vi "read_raw_dataV3.0_timestamp.vi"() -> ()   [LabVIEW 2017]
uses:
  <vilib>/Utility/file.llb/Read Delimited Spreadsheet (I64).vi
  <vilib>/Utility/file.llb/Write Delimited Spreadsheet (DBL).vi
  <vilib>/Utility/file.llb/Write Delimited Spreadsheet (I64).vi
  <vilib>/Utility/file.llb/Write Delimited Spreadsheet (string).vi
panel:
  out "offset past number 3":i32=1
  out "offset past number 2":i32=46
  out "offset past number":i32=15
  out "hex integer string 2":string="15"
  out "hex integer string":string="1"
  out "substring 5":string
  out "substring 4":string
  out "substring 3":string="."
  out "substring 2":string="46"
  out "output 1":timestamp=timestamp(3800538946 s since 1904-01-01)
  in  "output 4":timestamp=timestamp(3800536645.628 s since 1904-01-01)
  out "Numeric":dbl=-33699.628
  in  "date/time string 4":string="  6/7/2024"
  out "date/time string 3":string="1:15:46  6/7/2024"
  in  "col":i32
  in  "file path (dialog if empty)":path=path "G:/tdc/2017/code_density_rom.mem"
  out "size(s)":i32[](array[numeric])=[2048, 128]
  out "Array":u32[][](array[numeric]) format="%x"
  out "cal":u32[][](graph)
  out "x/y":dbl=0.0025
  out "index":i32=1018
  out "time":dbl=636682692500.0 format="%.000f"
  in  "通道数量":i32=128
  out "fine":u64=356 format="%x"
  out "data 5":string
  in  "ch list":u16[](array[numeric])=[0, 1, 2, 3, 4, 5, 6, 7]
  in  "codeDensity":path=path "G:/tdc/2017/test_20240607_060014_codeDensity.csv"
  out "file path (dialog if empty) 2":path=path "G:/tdc/2017/test_20240607_060014.txt"
  out "ip":u64=35 format="%x"
  out "data 9":string="#"
  out "result string":string="test_20240607_060014"
  out "sent number":u64=1000 format="%x"
  out "trigger number":u64=257 format="%x"
  out "data 8":string
  out "data 7":string
  out "data":u64[](array[numeric])=[35, 1, 1000, 257, 41715683595775000] format="%x"
  out "data 2":string
  out "data 4":string
  out "coarse time":u64=254673077 format="%x"
  out "error out":errorcluster
  out "substring":string=""
  out "number 3":u32
  out "channel number":u64=1 format="%x"
  in  "channel":u64
  out "data 6":string
  out "data 3":string="Z"
  in  "dat file (use dialog)":path=path "G:/tdc/2017/test_20240607_060014.dat"
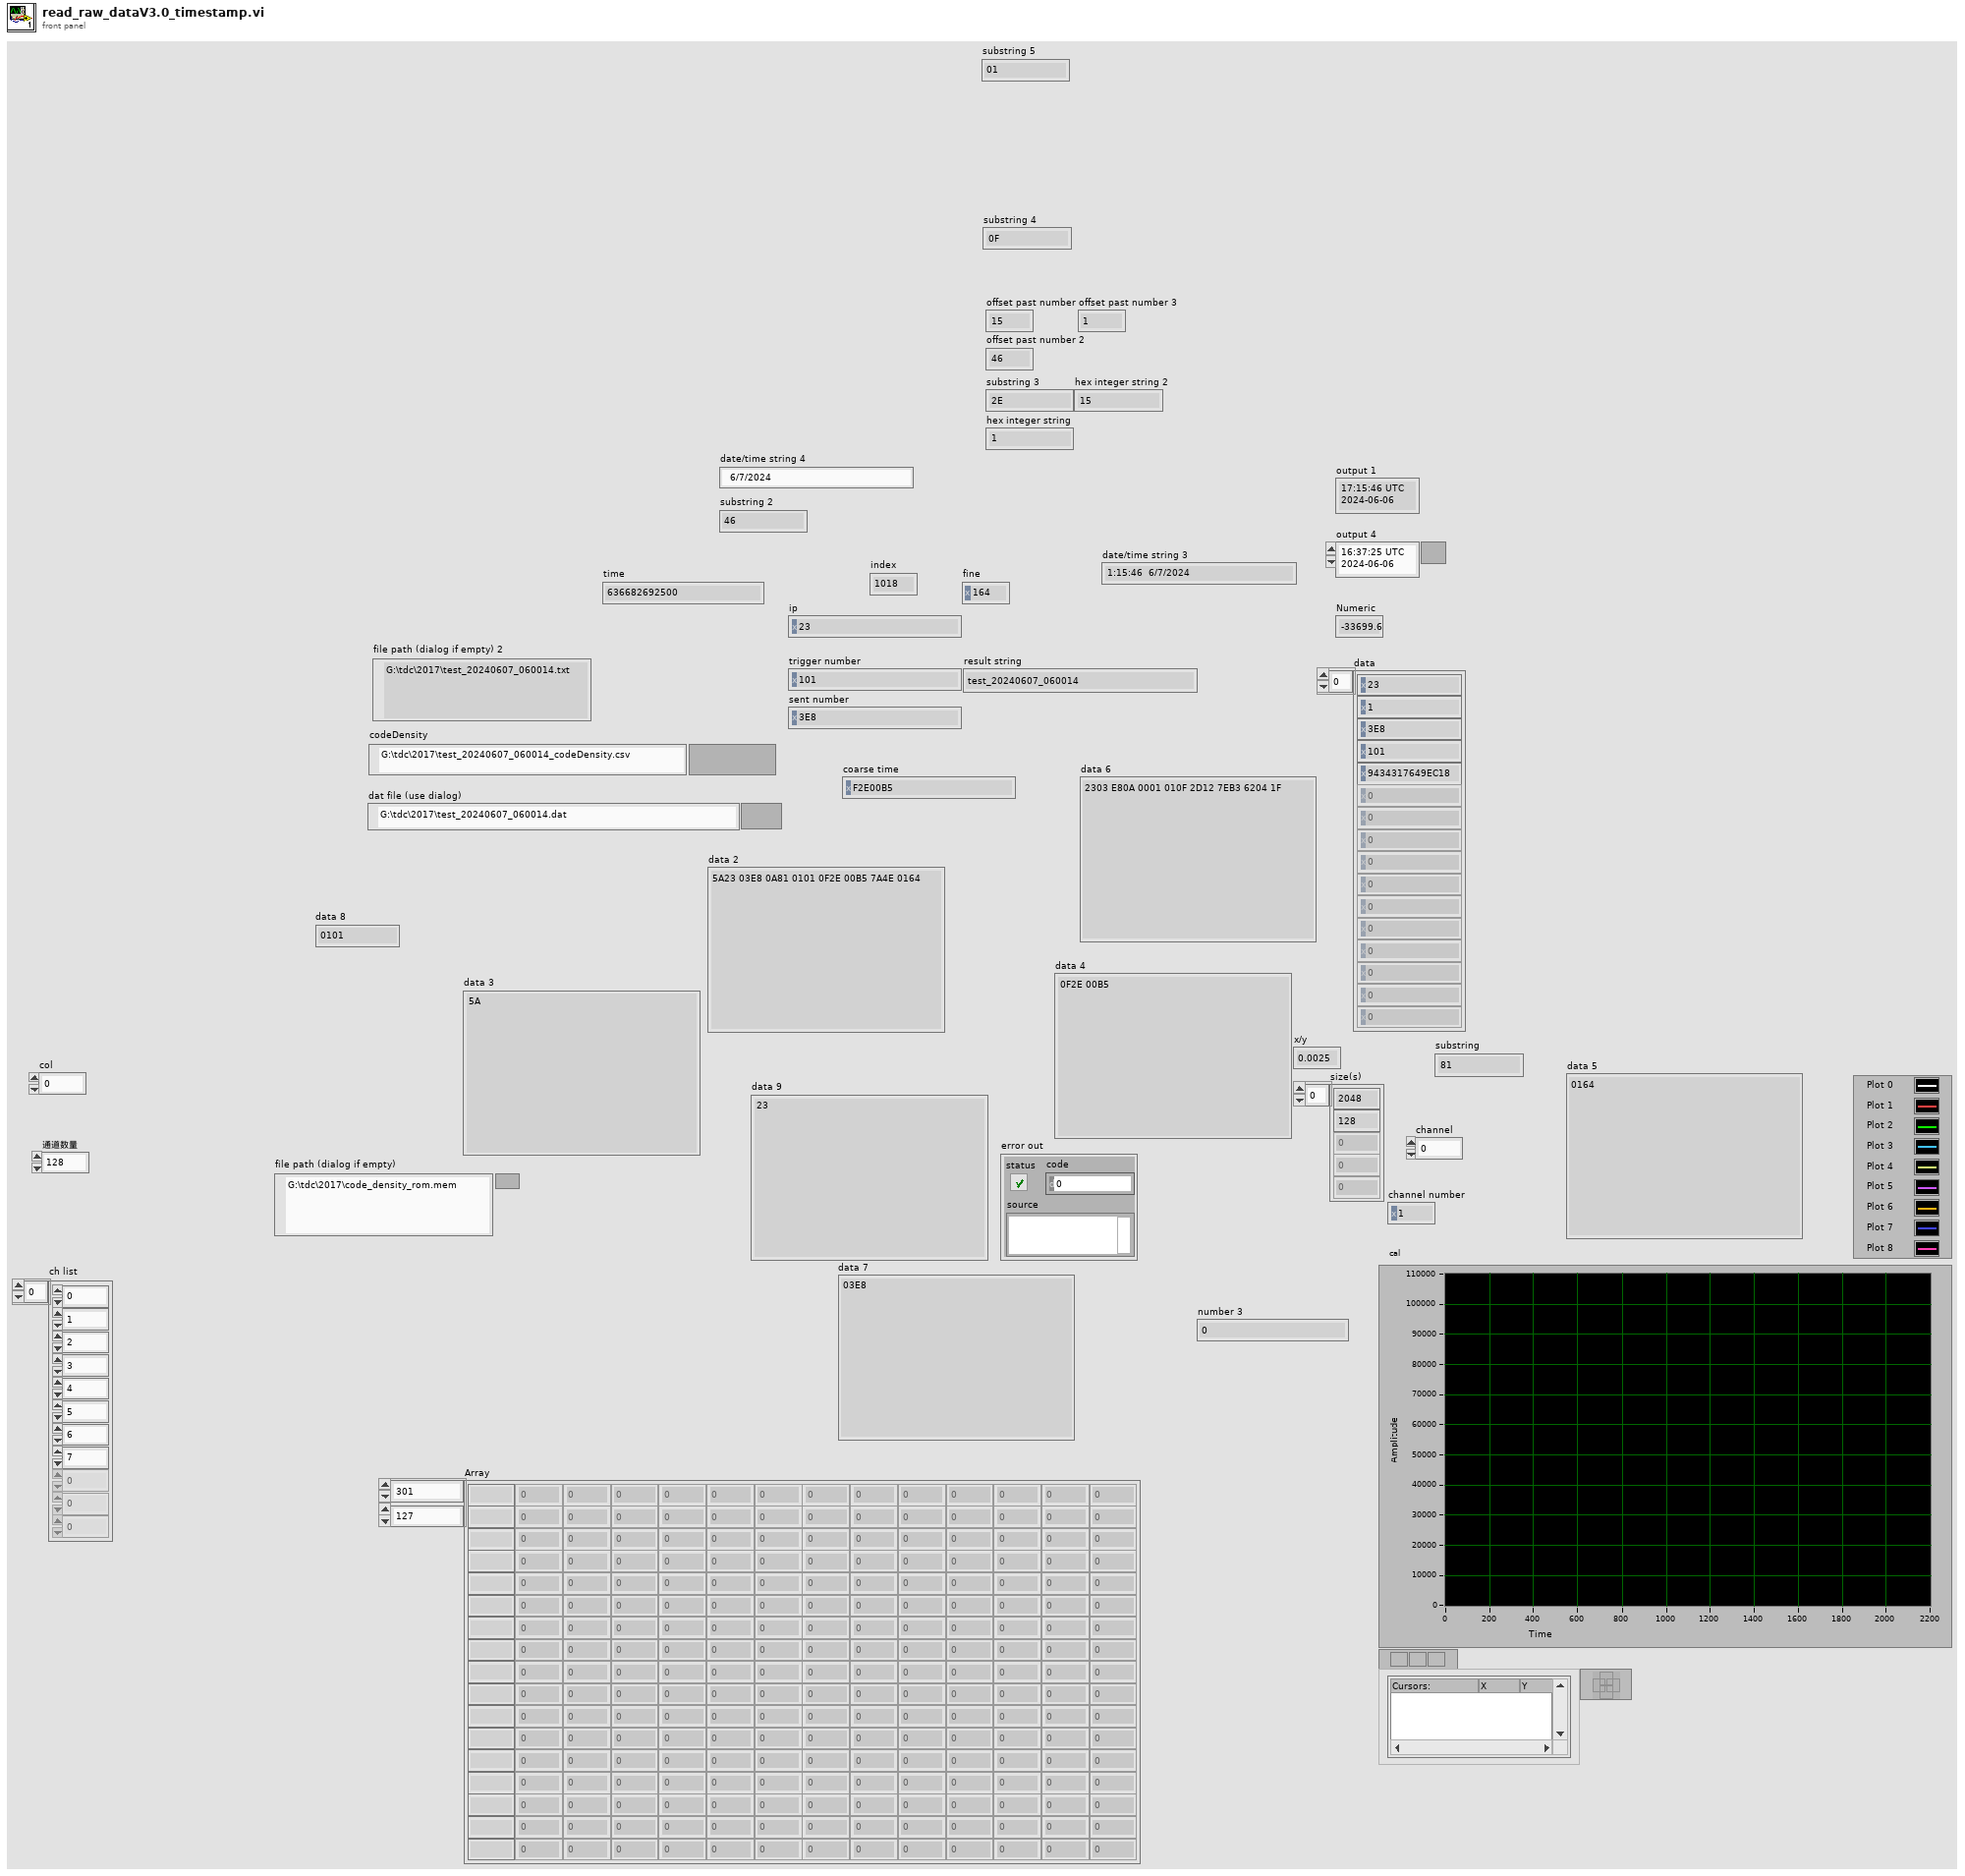
[diagram p1: front panel]
types:
  T1 = enum16{"open", "replace", "create", "open or create", "replace or create", "replace or create with confirmation"}
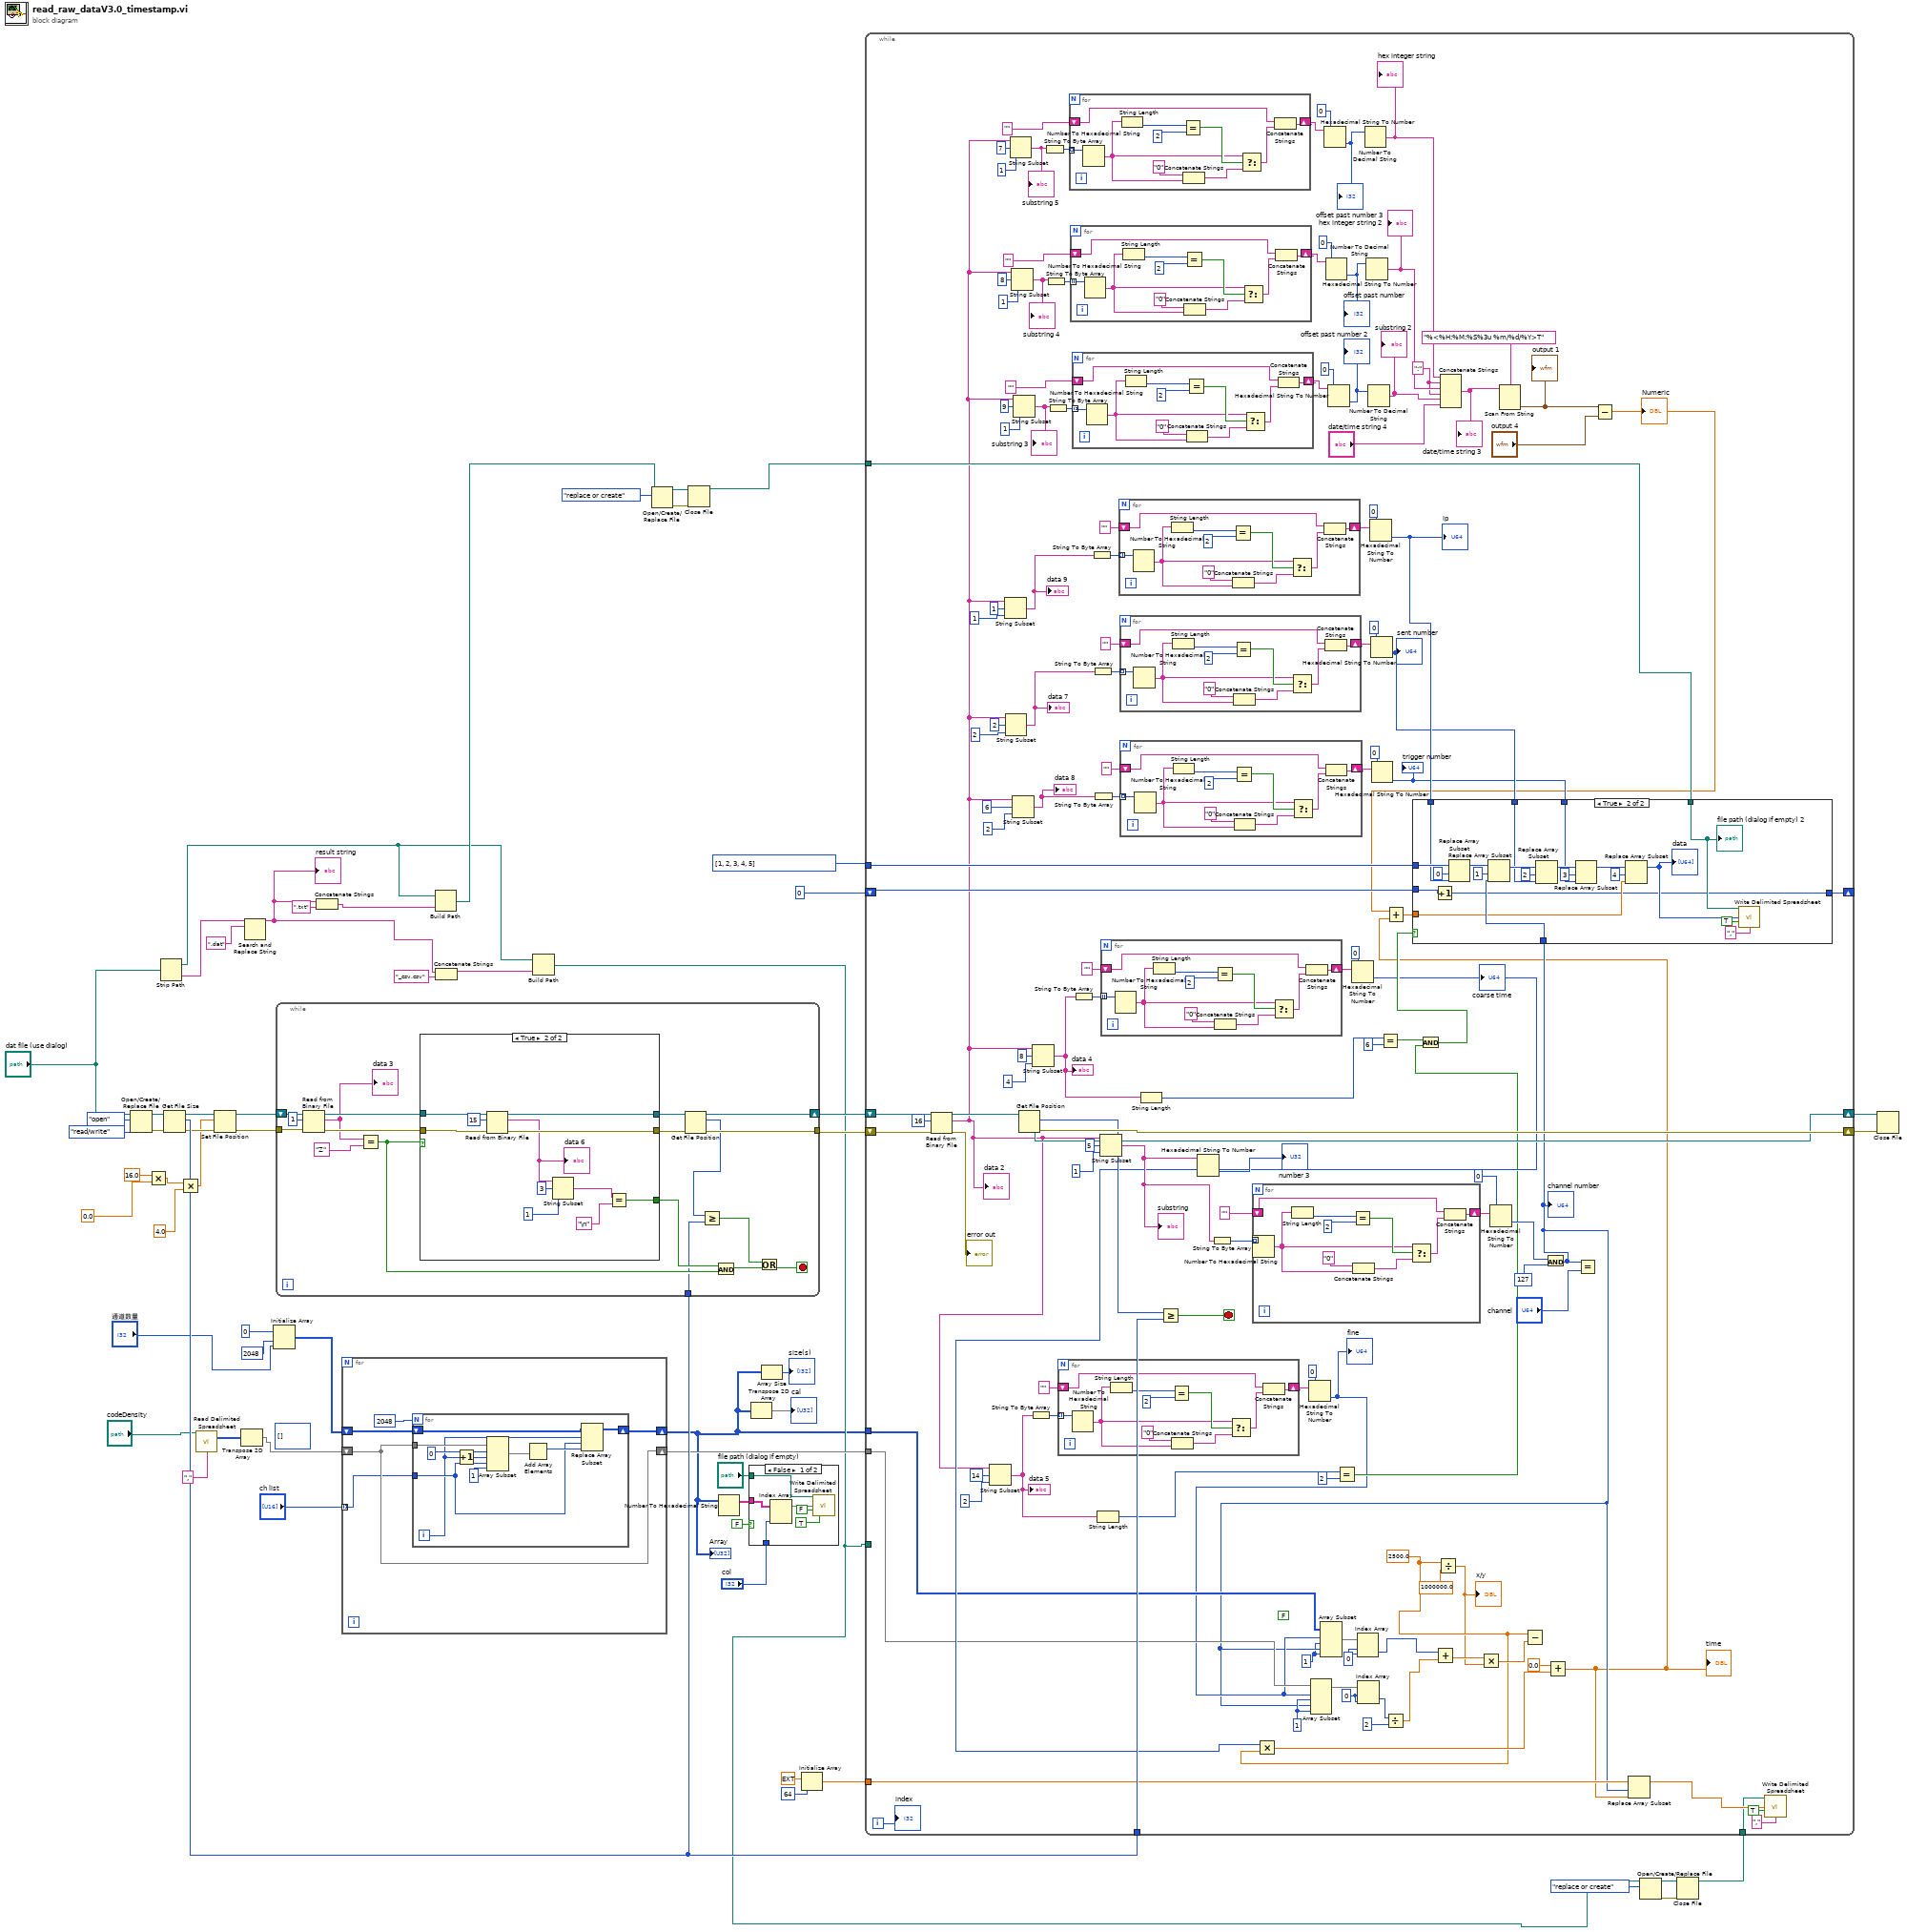
[diagram p0: block diagram]
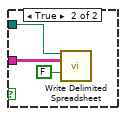
[diagram p2: hidden frame]
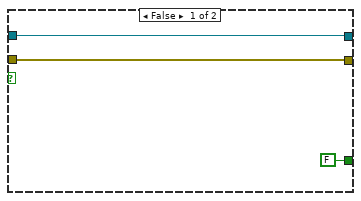
[diagram p4: hidden frame]
diagram:
  (unwired) i64[][] []
  n1 = Open/Create/Replace File(file path (use dialog)="dat file (use dialog)", operation (0:open)=T1."open", access (0:read/write)=enum16{"read/write", "read-only", "write-only"}."read/write") -> (refnum out=w59:refnum<file>, error out=w54:errorcluster)  [unwired: 3 in, 1 out]
  n2 = Multiply(x=16.0, y=0.0) -> (x*y=w20:dbl)
  n3 = Strip Path(path="dat file (use dialog)") -> (stripped path=w9:path, name=w47:string)
  n4 = Get File Size(file=w59, error in=w54) -> (refnum out=w26:refnum<file>, size (in bytes)=w49:i64, 0:w24:errorcluster)
  n5 = Multiply(x=w20, y=4.0) -> (x*y=w18:dbl)
  n6 = call-poly <vilib>:"Read Delimited Spreadsheet.vi"("file path (dialog if empty)"="codeDensity", "delimiter (\\t)"="," ("delimiter (\\t)")) -> ("all rows"=w43:i64[][])  [unwired: 8 in, 5 out]
  n7 = Set File Position(offset (in bytes) (0)=w18, refnum=w26, error in=w24) -> (refnum out=w25:refnum<file>, error out=w23:errorcluster)  [unwired: 1 in]
  n8 = Transpose 2D Array(2D array=w43) -> (transposed array=w31:i64[][])
  n9 = Search and Replace String(input string=w47, search string=".dat") -> (result string=w11:string)  [unwired: 6 in, 3 out]
  "result string" <- w11
  n10 = Initialize Array(u32 0 ("element"), 2048 ("dimension size"), "通道数量") -> (w32:u32[][])
  n11 = while {
    tunnel: w23 -> [w76]
    shift-right: [w64] -> w55
    shift-left: w25 -> [w77]
    tunnel: [w65] -> w56
    tunnel: w49 -> [w63]
    stop <- w61 stop-if-true
    n12 = Read from Binary File(8:w76, 10:1 ("count (1)"), 11:w77) -> (0:w72:errorcluster, 2:w70:string, 3:w73:refnum<file>)  [unwired: 3 in, 1 out]
    "data 3" <- w70
    n13 = Equal?(x=w70, y="Z") -> (x = y?=w67:bool)
    n14 = case shown="True" w67 {
      tunnel: w73 -> [w80 w91]
      tunnel: w72 -> [w79 w90]
      tunnel: [w80 w88] -> w71
      tunnel: [w79 w87] -> w66
      tunnel: [FALSE w81] -> w68
      frame False {
      }
      frame True {
        n15 = Read from Binary File(8:w90, 10:15 ("count (1)"), 11:w91) -> (0:w87:errorcluster, 2:w84:string, 3:w88:refnum<file>)  [unwired: 3 in, 1 out]
        "data 6" <- w84
        n16 = String Subset(string=w84, offset (0)=3, length (rest)=1 ("length (rest)")) -> (substring=w83:string)
        n17 = Equal?(x=w83, y="\n") -> (x = y?=w81:bool)
      }
    }
    n18 = Get File Position(4:w66, 7:w71) -> (0:w65:errorcluster, 2:w62:i64, 3:w64:refnum<file>)
    n19 = Greater Or Equal?(x=w62, y=w63) -> (x >= y?=w60:bool)
    n20 = Compound Arithmetic op=AND(w68, w67) -> (w69:bool)
    n21 = Or(x=w60, y=w69) -> (x .or. y?=w61:bool)
  }
  n22 = Concatenate Strings(w11, ".txt" ("string")) -> (w44:string)
  n23 = for {
    shift-right: [w94] -> w4
    shift-left: w32 -> [w95]
    shift-right: [w93] -> w39
    shift-left: w31 -> [w93]
    tunnel: "ch list" -> [w92] mode=indexing
    n24 = for {
      N: 2048 -> [_]
      tunnel: w93 -> [w106]
      tunnel: w92 -> [w99]
      shift-right: [w101] -> w94
      shift-left: w95 -> [w102]
      i -> [w98]
      n25 = Increment(x=w98) -> (x+1=w97:i32)
      n26 = Array Subset(array=w106, index (row)=0 ("索引"), length (row)=w97, index (col)=w99, length (col)=1 ("长度")) -> (w103:i64[][])
      n27 = Add Array Elements(numeric array=w103) -> (sum=w100:i64)
      n28 = Replace Array Subset(array=w102, new element=w100, index (row)=w98, index (col)=w99) -> (w101:u32[][])
    }
  }
  "Array" <- w4
  n29 = Build Path(base path=w9, name or relative path=w44) -> (appended path=w14:path)
  n30 = Concatenate Strings(w11, "_csv.csv" ("string")) -> (w10:string)
  n31 = Build Path(base path=w9, name or relative path=w10) -> (appended path=w8:path)
  n32 = Open/Create/Replace File(file path (use dialog)=w14, operation (0:open)=T1."replace or create") -> (refnum out=w15:refnum<file>, error out=w16:errorcluster)  [unwired: 4 in, 1 out]
  n33 = Close File(refnum=w15, error in=w16) -> (path=w13:path)  [unwired: 1 out]
  n34 = Number To Hexadecimal String(2:w4) -> (0:w3:string[][])  [unwired: 1 in]
  n35 = case shown="False" FALSE {
    tunnel: "file path (dialog if empty)" -> [w111 w115]
    tunnel: w3 -> [w110 w113]
    tunnel: "col" -> [w108 _]
    frame False {
      n36 = Index Array(array=w110, index (col)=w108) -> (element=w109:string[])  [unwired: 1 in]
      n37 = call-poly <vilib>:"Write Delimited Spreadsheet.vi"("file path (dialog if empty)"=w111, "1D data"=w109, "append to file? (new file:F)"=FALSE, "transpose? (no:F)"=TRUE) -> ()  [unwired: 10 in, 2 out]
    }
    frame True {
      n38 = call-poly <vilib>:"Write Delimited Spreadsheet.vi"("file path (dialog if empty)"=w115, "2D data"=w113, "append to file? (new file:F)"=FALSE) -> ()  [unwired: 11 in, 2 out]
    }
  }
  n39 = Transpose 2D Array(2D array=w4) -> (transposed array=→"cal":u32[][])
  n40 = Array Size(array=w4) -> (size(s)=→"size(s)":i32[])
  n41 = Initialize Array(ext 0.0 ("element"), 64 ("dimension size")) -> (w36:ext[])
  n42 = Open/Create/Replace File(file path (use dialog)=w8, operation (0:open)=T1."replace or create") -> (refnum out=w28:refnum<file>, error out=w29:errorcluster)  [unwired: 4 in, 1 out]
  n43 = Close File(refnum=w28, error in=w29) -> (path=w27:path)  [unwired: 1 out]
  n44 = while {
    shift-right: [w245] -> w53
    shift-left: w55 -> [w249]
    shift-right: [w247] -> w52
    shift-left: w56 -> [w250]
    tunnel: w49 -> [w243]
    shift-right: [w191] -> _
    shift-left: 0 ("length (rest)") -> [w222]
    tunnel: w13 -> [w192]
    tunnel: u64[] [1, 2, 3, 4, 5] -> [w221]
    tunnel: w4 -> [w166]
    tunnel: w39 -> [w167]
    tunnel: w36 -> [w162]
    tunnel: w27 -> [w155]
    tunnel: w8 -> [_]
    i -> [w154]
    stop <- w242 stop-if-true
    w117 = ":" ("string")
    w156 = 0 ("index (row)")
    w158 = 1 ("长度")
    w169 = 2500.0 ("x")
    (unwired) FALSE
    w182 = 0 ("索引 (行)")
    w184 = 1 ("长度")
    n45 = Read from Binary File(8:w250, 10:16 ("count (1)"), 11:w249) -> (0:→"error out":errorcluster, 2:w124:string, 3:w246:refnum<file>)  [unwired: 3 in, 1 out]
    "data 2" <- w124
    n46 = String Subset(string=w124, offset (0)=14, length (rest)=2 ("length (rest)")) -> (substring=w173:string)
    "data 5" <- w173
    n47 = String Subset(string=w124, offset (0)=1, length (rest)=1 ("length (rest)")) -> (substring=w202:string)
    "data 9" <- w202
    n48 = String Subset(string=w124, offset (0)=2, length (rest)=2 ("length (rest)")) -> (substring=w203:string)
    "data 7" <- w203
    n49 = String Subset(string=w124, offset (0)=7, length (rest)=1 ("length (rest)")) -> (substring=w125:string)
    "substring 5" <- w125
    n50 = String Subset(string=w124, offset (0)=8, length (rest)=1 ("length (rest)")) -> (substring=w138:string)
    "substring 4" <- w138
    n51 = String Subset(string=w124, offset (0)=6, length (rest)=2 ("length (rest)")) -> (substring=w208:string)
    "data 8" <- w208
    n52 = String Subset(string=w124, offset (0)=9, length (rest)=1 ("length (rest)")) -> (substring=w139:string)
    "substring 3" <- w139
    n53 = Get File Position(7:w246) -> (0:w247:errorcluster, 2:w244:i64, 3:w245:refnum<file>)  [unwired: 1 in]
    n54 = String To Byte Array(string=w173) -> (unsigned byte array=w176:u8[])
    n55 = String Subset(string=w124, offset (0)=8, length (rest)=4 ("length (rest)")) -> (substring=w219:string)
    "data 4" <- w219
    n56 = String To Byte Array(string=w125) -> (unsigned byte array=w128:u8[])
    n57 = String To Byte Array(string=w138) -> (unsigned byte array=w135:u8[])
    n58 = String To Byte Array(string=w139) -> (unsigned byte array=w142:u8[])
    n59 = for {
      shift-right: [w289] -> w175
      shift-left: "" ("format string") -> [w286]
      tunnel: w176 -> [w290] mode=indexing
      n60 = Number To Hexadecimal String(2:w290) -> (0:w282:string)  [unwired: 1 in]
      n61 = String Length(string=w282) -> (length=w288:i32)
      n62 = Equal?(x=w288, y=2) -> (x = y?=w285:bool)
      n63 = Concatenate Strings("0" ("format string"), w282) -> (w284:string)
      n64 = Select(t=w282, s=w285, f=w284) -> (s? t:f=w281:string)
      n65 = Concatenate Strings(w286, w281) -> (w289:string)
    }
    n66 = for {
      shift-right: [w259] -> w127
      shift-left: "" ("format string") -> [w256]
      tunnel: w128 -> [w260] mode=indexing
      n67 = Number To Hexadecimal String(2:w260) -> (0:w252:string)  [unwired: 1 in]
      n68 = String Length(string=w252) -> (length=w258:i32)
      n69 = Equal?(x=w258, y=2) -> (x = y?=w255:bool)
      n70 = Concatenate Strings("0" ("format string"), w252) -> (w254:string)
      n71 = Select(t=w252, s=w255, f=w254) -> (s? t:f=w251:string)
      n72 = Concatenate Strings(w256, w251) -> (w259:string)
    }
    n73 = for {
      shift-right: [w269] -> w136
      shift-left: "" ("format string") -> [w266]
      tunnel: w135 -> [w270] mode=indexing
      n74 = Number To Hexadecimal String(2:w270) -> (0:w262:string)  [unwired: 1 in]
      n75 = String Length(string=w262) -> (length=w268:i32)
      n76 = Equal?(x=w268, y=2) -> (x = y?=w265:bool)
      n77 = Concatenate Strings("0" ("format string"), w262) -> (w264:string)
      n78 = Select(t=w262, s=w265, f=w264) -> (s? t:f=w261:string)
      n79 = Concatenate Strings(w266, w261) -> (w269:string)
    }
    n80 = for {
      shift-right: [w279] -> w141
      shift-left: "" ("format string") -> [w276]
      tunnel: w142 -> [w280] mode=indexing
      n81 = Number To Hexadecimal String(2:w280) -> (0:w272:string)  [unwired: 1 in]
      n82 = String Length(string=w272) -> (length=w278:i32)
      n83 = Equal?(x=w278, y=2) -> (x = y?=w275:bool)
      n84 = Concatenate Strings("0" ("format string"), w272) -> (w274:string)
      n85 = Select(t=w272, s=w275, f=w274) -> (s? t:f=w271:string)
      n86 = Concatenate Strings(w276, w271) -> (w279:string)
    }
    n87 = String To Byte Array(string=w219) -> (unsigned byte array=w238:u8[])
    n88 = String To Byte Array(string=w202) -> (unsigned byte array=w199:u8[])
    n89 = String To Byte Array(string=w203) -> (unsigned byte array=w206:u8[])
    n90 = String To Byte Array(string=w208) -> (unsigned byte array=w210:u8[])
    n91 = String Length(string=w173) -> (length=w172:i32)
    n92 = String Subset(string=w124, offset (0)=5, length (rest)=1 ("length (rest)")) -> (substring=w225:string)
    "substring" <- w225
    n93 = for {
      shift-right: [w361] -> w237
      shift-left: "" ("format string") -> [w358]
      tunnel: w238 -> [w362] mode=indexing
      n94 = Number To Hexadecimal String(2:w362) -> (0:w354:string)  [unwired: 1 in]
      n95 = String Length(string=w354) -> (length=w360:i32)
      n96 = Equal?(x=w360, y=2) -> (x = y?=w357:bool)
      n97 = Concatenate Strings("0" ("format string"), w354) -> (w356:string)
      n98 = Select(t=w354, s=w357, f=w356) -> (s? t:f=w353:string)
      n99 = Concatenate Strings(w358, w353) -> (w361:string)
    }
    n100 = for {
      shift-right: [w299] -> w200
      shift-left: "" ("format string") -> [w296]
      tunnel: w199 -> [w300] mode=indexing
      n101 = Number To Hexadecimal String(2:w300) -> (0:w292:string)  [unwired: 1 in]
      n102 = String Length(string=w292) -> (length=w298:i32)
      n103 = Equal?(x=w298, y=2) -> (x = y?=w295:bool)
      n104 = Concatenate Strings("0" ("format string"), w292) -> (w294:string)
      n105 = Select(t=w292, s=w295, f=w294) -> (s? t:f=w291:string)
      n106 = Concatenate Strings(w296, w291) -> (w299:string)
    }
    n107 = for {
      shift-right: [w309] -> w205
      shift-left: "" ("format string") -> [w306]
      tunnel: w206 -> [w310] mode=indexing
      n108 = Number To Hexadecimal String(2:w310) -> (0:w302:string)  [unwired: 1 in]
      n109 = String Length(string=w302) -> (length=w308:i32)
      n110 = Equal?(x=w308, y=2) -> (x = y?=w305:bool)
      n111 = Concatenate Strings("0" ("format string"), w302) -> (w304:string)
      n112 = Select(t=w302, s=w305, f=w304) -> (s? t:f=w301:string)
      n113 = Concatenate Strings(w306, w301) -> (w309:string)
    }
    n114 = for {
      shift-right: [w319] -> w211
      shift-left: "" ("format string") -> [w316]
      tunnel: w210 -> [w320] mode=indexing
      n115 = Number To Hexadecimal String(2:w320) -> (0:w312:string)  [unwired: 1 in]
      n116 = String Length(string=w312) -> (length=w318:i32)
      n117 = Equal?(x=w318, y=2) -> (x = y?=w315:bool)
      n118 = Concatenate Strings("0" ("format string"), w312) -> (w314:string)
      n119 = Select(t=w312, s=w315, f=w314) -> (s? t:f=w311:string)
      n120 = Concatenate Strings(w316, w311) -> (w319:string)
    }
    n121 = String Length(string=w219) -> (length=w217:i32)
    n122 = Greater Or Equal?(x=w244, y=w243) -> (x >= y?=w242:bool)
    n123 = Hexadecimal String To Number(string=w225) -> (number=→"number 3":u32)  [unwired: 2 in, 1 out]
    n124 = String To Byte Array(string=w225) -> (unsigned byte array=w228:u8[])
    n125 = for {
      shift-right: [w351] -> w227
      shift-left: "" ("format string") -> [w348]
      tunnel: w228 -> [w352] mode=indexing
      n126 = Number To Hexadecimal String(2:w352) -> (0:w344:string)  [unwired: 1 in]
      n127 = String Length(string=w344) -> (length=w350:i32)
      n128 = Equal?(x=w350, y=2) -> (x = y?=w347:bool)
      n129 = Concatenate Strings("0" ("format string"), w344) -> (w346:string)
      n130 = Select(t=w344, s=w347, f=w346) -> (s? t:f=w343:string)
      n131 = Concatenate Strings(w348, w343) -> (w351:string)
    }
    n132 = Hexadecimal String To Number(string=w175, default (0uL)=u64 0 ("default (0 U32)")) -> (number=w164:u64)  [unwired: 1 in, 1 out]
    "fine" <- w164
    n133 = Hexadecimal String To Number(string=w127, default (0uL)=u64 0 ("default (0 U32)")) -> (number=w120:u64)  [unwired: 1 in, 1 out]
    "offset past number 3" <- w120
    n134 = Hexadecimal String To Number(string=w136, default (0uL)=u64 0 ("default (0 U32)")) -> (number=w121:u64)  [unwired: 1 in, 1 out]
    "offset past number" <- w121
    n135 = Hexadecimal String To Number(string=w141, default (0uL)=u64 0 ("default (0 U32)")) -> (number=w122:u64)  [unwired: 1 in, 1 out]
    "offset past number 2" <- w122
    n136 = Equal?(x=w172, y=2) -> (x = y?=w165:bool)
    n137 = Hexadecimal String To Number(string=w237, default (0uL)=u64 0 ("default (0 U32)")) -> (number=w170:u64)  [unwired: 1 in, 1 out]
    "coarse time" <- w170
    n138 = Multiply(x=w170, y=w169) -> (x*y=w186:dbl)
    n139 = Number To Decimal String(number=w120) -> (decimal integer string=w119:string)  [unwired: 1 in]
    "hex integer string" <- w119
    n140 = Number To Decimal String(number=w121) -> (decimal integer string=w123:string)  [unwired: 1 in]
    "hex integer string 2" <- w123
    n141 = Number To Decimal String(number=w122) -> (decimal integer string=w118:string)  [unwired: 1 in]
    "substring 2" <- w118
    n142 = Hexadecimal String To Number(string=w200, default (0uL)=u64 0 ("default (0 U32)")) -> (number=w195:u64)  [unwired: 1 in, 1 out]
    "ip" <- w195
    n143 = Hexadecimal String To Number(string=w205, default (0uL)=u64 0 ("default (0 U32)")) -> (number=w194:u64)  [unwired: 1 in, 1 out]
    "sent number" <- w194
    n144 = Hexadecimal String To Number(string=w211, default (0uL)=u64 0 ("default (0 U32)")) -> (number=w193:u64)  [unwired: 1 in, 1 out]
    "trigger number" <- w193
    n145 = Equal?(x=w217, y=6) -> (x = y?=w218:bool)
    n146 = And(x=w218, y=w165) -> (x .and. y?=w215:bool)
    n147 = Divide(x=w169, y=1000000.0) -> (x/y=w168:dbl)
    "x/y" <- w168
    n148 = Concatenate Strings(w119, w117, w123, w117, w118, "date/time string 4") -> (w150:string)
    "date/time string 3" <- w150
    n149 = Hexadecimal String To Number(string=w227, default (0uL)=u64 0 ("default (0 U32)")) -> (number=w224:u64)  [unwired: 1 in, 1 out]
    n150 = Scan From String(format string="%<%H:%M:%S%3u %m/%d/%Y>T", input string=w150) -> (output 1=w147:timestamp)  [unwired: 3 in, 3 out]
    "output 1" <- w147
    n151 = And(x=w224, y=u64 127 ("default (0 U32)")) -> (x .and. y?=w161:u64)
    "channel number" <- w161
    n152 = Array Subset(array=w167, index (row)=w164, length (row)=w184, index (col)=w161, length (col)=w184) -> (w183:i64[][])
    n153 = Array Subset(array=w166, index (row)=w164, length (row)=w158, index (col)=w161, length (col)=w158) -> (w157:u32[][])
    n154 = Index Array(array=w157, index (row)=w156, index (col)=w156) -> (element=w188:u32)
    n155 = Index Array(array=w183, index (row)=w182, index (col)=w182) -> (element=w181:i64)
    n156 = Divide(x=w181, y=u32 2) -> (x/y=w185:dbl)
    n157 = Add(x=w188, y=w185) -> (x+y=w187:dbl)
    n158 = Multiply(x=w187, y=w168) -> (x*y=w180:dbl)
    n159 = Subtract(x=w169, y=w180) -> ()  [unwired: 1 out]
    n160 = Add(x=0.0, y=w186) -> (x+y=w146:dbl)
    "time" <- w146
    n161 = Equal?(x=w161, y="channel") -> ()  [unwired: 1 out]
    n162 = Subtract(x=w147, y="output 4") -> (x-y=w144:dbl)
    "Numeric" <- w144
    n163 = Add(x=w144, y=w146) -> (x+y=w145:dbl)
    n164 = case shown="True" w215 {
      tunnel: w222 -> [w321 w324]
      tunnel: w221 -> [_ w342]
      tunnel: w145 -> [_ w325]
      tunnel: w195 -> [_ w340]
      tunnel: w194 -> [_ w332]
      tunnel: w193 -> [_ w333]
      tunnel: w161 -> [_ w331]
      tunnel: w192 -> [_ w329]
      tunnel: [w321 w323] -> w191
      frame False {
      }
      frame True {
        n165 = Increment(x=w324) -> (x+1=w323:i32)
        n166 = Replace Array Subset(array=w342, new element=w340, index=0) -> (w339:u64[])
        n167 = Replace Array Subset(array=w339, new element=w331, index=1) -> (w334:u64[])
        n168 = Replace Array Subset(array=w334, new element=w332, index=2) -> (w336:u64[])
        n169 = Replace Array Subset(array=w336, new element=w333, index=3) -> (w327:u64[])
        n170 = Replace Array Subset(array=w327, new element=w325, index=4) -> (w326:u64[])
        "data" <- w326
        n171 = call-poly <vilib>:"Write Delimited Spreadsheet.vi"("file path (dialog if empty)"=w329, "1D data"=w326, "append to file? (new file:F)"=TRUE, "delimiter (\\t)"="," ("delimiter (\\t)")) -> ()  [unwired: 10 in, 2 out]
        "file path (dialog if empty) 2" <- w329
      }
    }
    n172 = Replace Array Subset(array=w162, new element=w146, index=w161) -> (w160:ext[])
    n173 = call-poly <vilib>:"Write Delimited Spreadsheet.vi"("file path (dialog if empty)"=w155, "1D data"=w160, "append to file? (new file:F)"=TRUE, "delimiter (\\t)"="," ("delimiter (\\t)")) -> ()  [unwired: 10 in, 2 out]
    "index" <- w154
  }
  n174 = Close File(refnum=w53, error in=w52) -> ()  [unwired: 2 out]
